vi "XLP80_Action_UpdateWriteB_newState.vi"(8 "err in":errorcluster, 10 "Function":string) -> (0 "err out":errorcluster)   [LabVIEW 2021]
uses:
  XLP80_FGlob/1886_FGlob_TDefs_Enum_FGlobItems.ctl
  XLP80_Globals/Globals_Settings_XLP80.vi
  XLP80_Globals/XLP80_Globals_Referenzen.vi
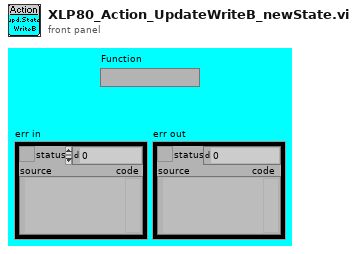
[diagram p1: front panel]
types:
  T1 = cluster{"Signal Name":string[], "Description":string[], "Unit":string[], "Default":dbl[], "Min":dbl[], "Max":dbl[], "Preconditions":bool[], "HV & Software":bool[], "Basis Funktion":bool[], "Power Management":bool[], "OperationMode":bool[], "Shutdown":bool[], "Alarm":bool[], "LogEnable":bool[]}
  T2 = typedef "1886_FGlob_TDefs_Enum_FGlobItems.ctl" = enum16{"Put one", "Put all", "Recall one", "Recall all"}
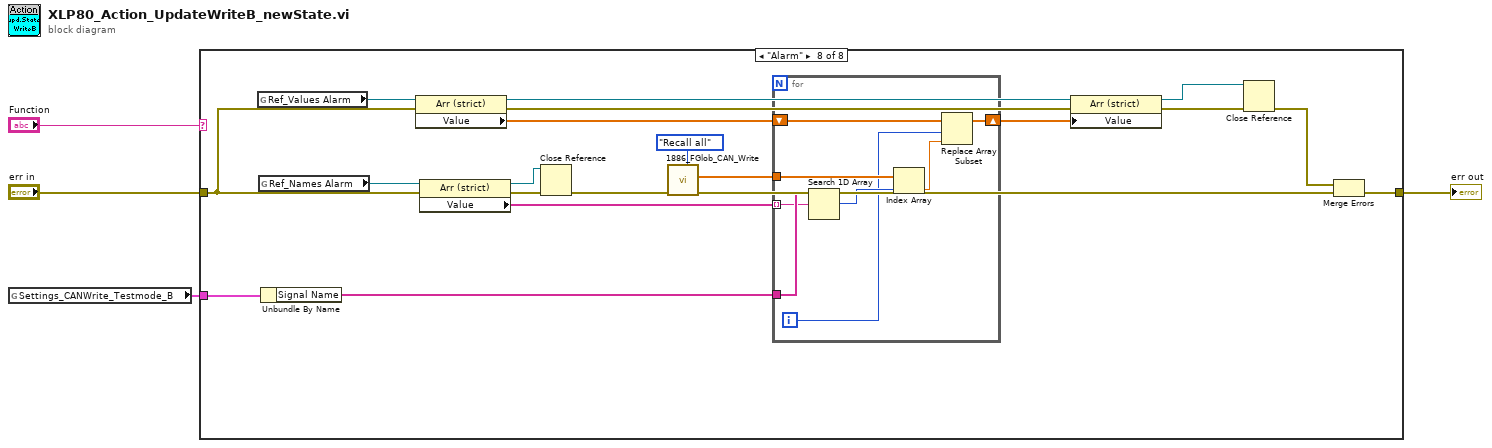
[diagram p0: block diagram]
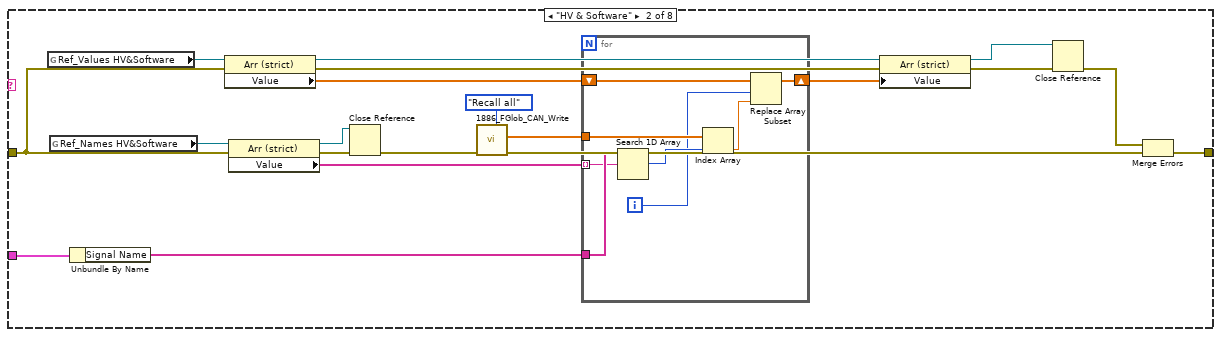
[diagram p3: hidden frame]
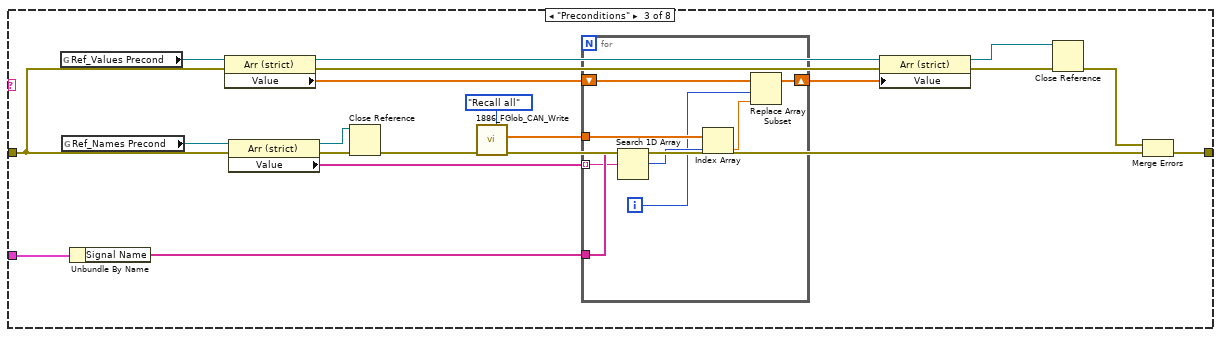
[diagram p4: hidden frame]
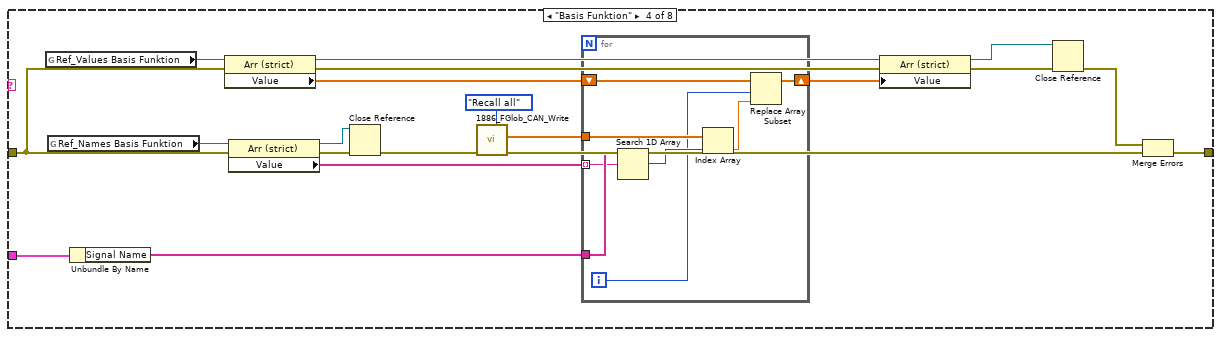
[diagram p5: hidden frame]
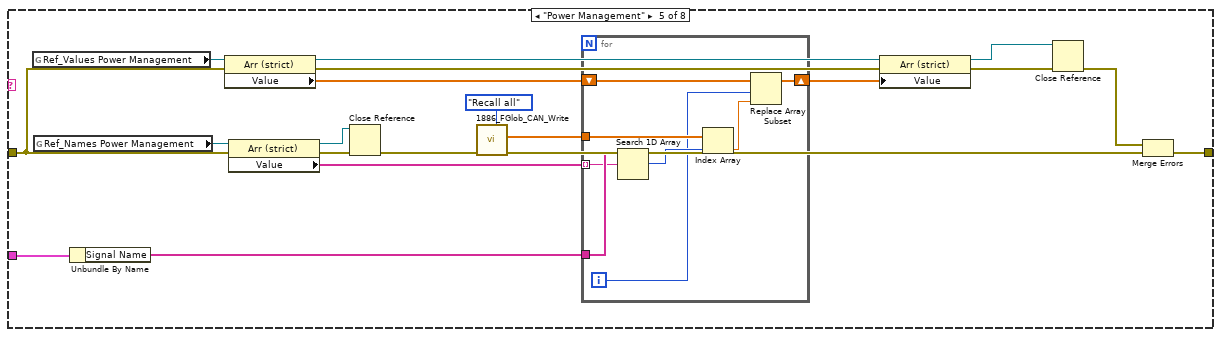
[diagram p6: hidden frame]
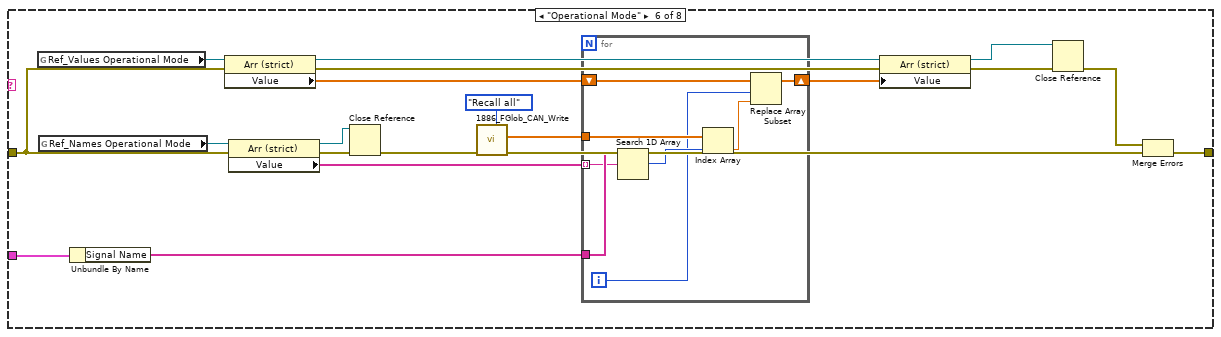
[diagram p7: hidden frame]
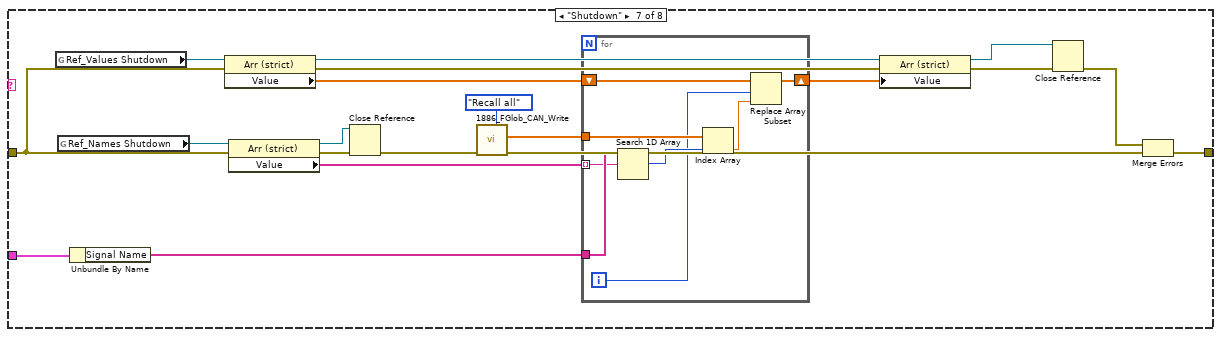
[diagram p8: hidden frame]
diagram:
  n1 = global read "Globals_Settings_XLP80.vi" "Settings_CANWrite_Testmode_B"() -> (w4:T1)
  n2 = case shown="\"Alarm\"" "Function" {
    tunnel: w4 -> [_ w19 w47 w75 w103 w131 w159 w187]
    tunnel: "err in" -> [w5 w18 w46 w74 w102 w130 w158 w186]
    tunnel: [w5 w21 w49 w77 w105 w133 w161 w189] -> w2
    frame Default {
    }
    frame "HV & Software" {
      n3 = global read "XLP80_Globals_Referenzen.vi" "Ref_Values HV&Software"() -> (w22:refnum<vi>)
      n4 = global read "XLP80_Globals_Referenzen.vi" "Ref_Names HV&Software"() -> (w23:refnum<vi>)
      n5 = Unbundle By Name(w19) -> ("Signal Name"=w15:string[])
      n6 = property class="Arr (strict)"(reference=w22, error in=w18) -> (reference out=w10:refnum<vi>, error out=w9:errorcluster, "Value"=w17:dbl[])
      n7 = property class="Arr (strict)"(reference=w23, error in=w18) -> (reference out=w24:refnum<vi>, error out=w25:errorcluster, "Value"=w16:string[])
      n8 = Close Reference(reference=w24, error in (no error)=w25) -> (error out=w14:errorcluster)
      n9 = call "1886_FGlob_CAN_Write.vi"("Function (Recall One)"=1886_FGlob_TDefs_Enum_FGlobItems."Recall all", "err in"=w14) -> ("err out"=w11:errorcluster, "AO Values OUT"=w12:dbl[])  [unwired: 7 in, 1 out]
      n10 = for {
        shift-right: [w26] -> w8
        shift-left: w17 -> [w31]
        tunnel: w16 -> [w32] mode=indexing
        tunnel: w15 -> [w33]
        tunnel: w12 -> [w30]
        i -> [w28]
        n11 = Search 1D Array(1D array=w33, element=w32) -> (index of element=w29:i32)  [unwired: 1 in]
        n12 = Index Array(array=w30, index=w29) -> (element=w27:dbl)
        n13 = Replace Array Subset(array=w31, new element=w27, index=w28) -> (w26:dbl[])
      }
      n14 = property class="Arr (strict)"(reference=w10, error in=w9, "Value"=w8) -> (reference out=w7:refnum<vi>, error out=w6:errorcluster)
      n15 = Close Reference(reference=w7, error in (no error)=w6) -> (error out=w20:errorcluster)
      n16 = Merge Errors(w20, w11) -> (w21:errorcluster)
    }
    frame "Preconditions" {
      n17 = global read "XLP80_Globals_Referenzen.vi" "Ref_Values Precond"() -> (w50:refnum<vi>)
      n18 = global read "XLP80_Globals_Referenzen.vi" "Ref_Names Precond"() -> (w51:refnum<vi>)
      n19 = Unbundle By Name(w47) -> ("Signal Name"=w43:string[])
      n20 = property class="Arr (strict)"(reference=w50, error in=w46) -> (reference out=w38:refnum<vi>, error out=w37:errorcluster, "Value"=w45:dbl[])
      n21 = property class="Arr (strict)"(reference=w51, error in=w46) -> (reference out=w52:refnum<vi>, error out=w53:errorcluster, "Value"=w44:string[])
      n22 = Close Reference(reference=w52, error in (no error)=w53) -> (error out=w42:errorcluster)
      n23 = call "1886_FGlob_CAN_Write.vi"("Function (Recall One)"=1886_FGlob_TDefs_Enum_FGlobItems."Recall all", "err in"=w42) -> ("err out"=w39:errorcluster, "AO Values OUT"=w40:dbl[])  [unwired: 7 in, 1 out]
      n24 = for {
        shift-right: [w54] -> w36
        shift-left: w45 -> [w59]
        tunnel: w44 -> [w60] mode=indexing
        tunnel: w43 -> [w61]
        tunnel: w40 -> [w58]
        i -> [w56]
        n25 = Search 1D Array(1D array=w61, element=w60) -> (index of element=w57:i32)  [unwired: 1 in]
        n26 = Index Array(array=w58, index=w57) -> (element=w55:dbl)
        n27 = Replace Array Subset(array=w59, new element=w55, index=w56) -> (w54:dbl[])
      }
      n28 = property class="Arr (strict)"(reference=w38, error in=w37, "Value"=w36) -> (reference out=w35:refnum<vi>, error out=w34:errorcluster)
      n29 = Close Reference(reference=w35, error in (no error)=w34) -> (error out=w48:errorcluster)
      n30 = Merge Errors(w48, w39) -> (w49:errorcluster)
    }
    frame "Basis Funktion" {
      n31 = global read "XLP80_Globals_Referenzen.vi" "Ref_Values Basis Funktion"() -> (w78:refnum<vi>)
      n32 = global read "XLP80_Globals_Referenzen.vi" "Ref_Names Basis Funktion"() -> (w79:refnum<vi>)
      n33 = Unbundle By Name(w75) -> ("Signal Name"=w71:string[])
      n34 = property class="Arr (strict)"(reference=w78, error in=w74) -> (reference out=w66:refnum<vi>, error out=w65:errorcluster, "Value"=w73:dbl[])
      n35 = property class="Arr (strict)"(reference=w79, error in=w74) -> (reference out=w80:refnum<vi>, error out=w81:errorcluster, "Value"=w72:string[])
      n36 = Close Reference(reference=w80, error in (no error)=w81) -> (error out=w70:errorcluster)
      n37 = call "1886_FGlob_CAN_Write.vi"("Function (Recall One)"=1886_FGlob_TDefs_Enum_FGlobItems."Recall all", "err in"=w70) -> ("err out"=w67:errorcluster, "AO Values OUT"=w68:dbl[])  [unwired: 7 in, 1 out]
      n38 = for {
        shift-right: [w82] -> w64
        shift-left: w73 -> [w87]
        tunnel: w72 -> [w88] mode=indexing
        tunnel: w71 -> [w89]
        tunnel: w68 -> [w86]
        i -> [w84]
        n39 = Search 1D Array(1D array=w89, element=w88) -> (index of element=w85:i32)  [unwired: 1 in]
        n40 = Index Array(array=w86, index=w85) -> (element=w83:dbl)
        n41 = Replace Array Subset(array=w87, new element=w83, index=w84) -> (w82:dbl[])
      }
      n42 = property class="Arr (strict)"(reference=w66, error in=w65, "Value"=w64) -> (reference out=w63:refnum<vi>, error out=w62:errorcluster)
      n43 = Close Reference(reference=w63, error in (no error)=w62) -> (error out=w76:errorcluster)
      n44 = Merge Errors(w76, w67) -> (w77:errorcluster)
    }
    frame "Power Management" {
      n45 = global read "XLP80_Globals_Referenzen.vi" "Ref_Values Power Management"() -> (w106:refnum<vi>)
      n46 = global read "XLP80_Globals_Referenzen.vi" "Ref_Names Power Management"() -> (w107:refnum<vi>)
      n47 = Unbundle By Name(w103) -> ("Signal Name"=w99:string[])
      n48 = property class="Arr (strict)"(reference=w106, error in=w102) -> (reference out=w94:refnum<vi>, error out=w93:errorcluster, "Value"=w101:dbl[])
      n49 = property class="Arr (strict)"(reference=w107, error in=w102) -> (reference out=w108:refnum<vi>, error out=w109:errorcluster, "Value"=w100:string[])
      n50 = Close Reference(reference=w108, error in (no error)=w109) -> (error out=w98:errorcluster)
      n51 = call "1886_FGlob_CAN_Write.vi"("Function (Recall One)"=1886_FGlob_TDefs_Enum_FGlobItems."Recall all", "err in"=w98) -> ("err out"=w95:errorcluster, "AO Values OUT"=w96:dbl[])  [unwired: 7 in, 1 out]
      n52 = for {
        shift-right: [w110] -> w92
        shift-left: w101 -> [w115]
        tunnel: w100 -> [w116] mode=indexing
        tunnel: w99 -> [w117]
        tunnel: w96 -> [w114]
        i -> [w112]
        n53 = Search 1D Array(1D array=w117, element=w116) -> (index of element=w113:i32)  [unwired: 1 in]
        n54 = Index Array(array=w114, index=w113) -> (element=w111:dbl)
        n55 = Replace Array Subset(array=w115, new element=w111, index=w112) -> (w110:dbl[])
      }
      n56 = property class="Arr (strict)"(reference=w94, error in=w93, "Value"=w92) -> (reference out=w91:refnum<vi>, error out=w90:errorcluster)
      n57 = Close Reference(reference=w91, error in (no error)=w90) -> (error out=w104:errorcluster)
      n58 = Merge Errors(w104, w95) -> (w105:errorcluster)
    }
    frame "Operational Mode" {
      n59 = global read "XLP80_Globals_Referenzen.vi" "Ref_Values Operational Mode"() -> (w134:refnum<vi>)
      n60 = global read "XLP80_Globals_Referenzen.vi" "Ref_Names Operational Mode"() -> (w135:refnum<vi>)
      n61 = Unbundle By Name(w131) -> ("Signal Name"=w127:string[])
      n62 = property class="Arr (strict)"(reference=w134, error in=w130) -> (reference out=w122:refnum<vi>, error out=w121:errorcluster, "Value"=w129:dbl[])
      n63 = property class="Arr (strict)"(reference=w135, error in=w130) -> (reference out=w136:refnum<vi>, error out=w137:errorcluster, "Value"=w128:string[])
      n64 = Close Reference(reference=w136, error in (no error)=w137) -> (error out=w126:errorcluster)
      n65 = call "1886_FGlob_CAN_Write.vi"("Function (Recall One)"=1886_FGlob_TDefs_Enum_FGlobItems."Recall all", "err in"=w126) -> ("err out"=w123:errorcluster, "AO Values OUT"=w124:dbl[])  [unwired: 7 in, 1 out]
      n66 = for {
        shift-right: [w138] -> w120
        shift-left: w129 -> [w143]
        tunnel: w128 -> [w144] mode=indexing
        tunnel: w127 -> [w145]
        tunnel: w124 -> [w142]
        i -> [w140]
        n67 = Search 1D Array(1D array=w145, element=w144) -> (index of element=w141:i32)  [unwired: 1 in]
        n68 = Index Array(array=w142, index=w141) -> (element=w139:dbl)
        n69 = Replace Array Subset(array=w143, new element=w139, index=w140) -> (w138:dbl[])
      }
      n70 = property class="Arr (strict)"(reference=w122, error in=w121, "Value"=w120) -> (reference out=w119:refnum<vi>, error out=w118:errorcluster)
      n71 = Close Reference(reference=w119, error in (no error)=w118) -> (error out=w132:errorcluster)
      n72 = Merge Errors(w132, w123) -> (w133:errorcluster)
    }
    frame "Shutdown" {
      n73 = global read "XLP80_Globals_Referenzen.vi" "Ref_Values Shutdown"() -> (w162:refnum<vi>)
      n74 = global read "XLP80_Globals_Referenzen.vi" "Ref_Names Shutdown"() -> (w163:refnum<vi>)
      n75 = Unbundle By Name(w159) -> ("Signal Name"=w155:string[])
      n76 = property class="Arr (strict)"(reference=w162, error in=w158) -> (reference out=w150:refnum<vi>, error out=w149:errorcluster, "Value"=w157:dbl[])
      n77 = property class="Arr (strict)"(reference=w163, error in=w158) -> (reference out=w164:refnum<vi>, error out=w165:errorcluster, "Value"=w156:string[])
      n78 = Close Reference(reference=w164, error in (no error)=w165) -> (error out=w154:errorcluster)
      n79 = call "1886_FGlob_CAN_Write.vi"("Function (Recall One)"=1886_FGlob_TDefs_Enum_FGlobItems."Recall all", "err in"=w154) -> ("err out"=w151:errorcluster, "AO Values OUT"=w152:dbl[])  [unwired: 7 in, 1 out]
      n80 = for {
        shift-right: [w166] -> w148
        shift-left: w157 -> [w171]
        tunnel: w156 -> [w172] mode=indexing
        tunnel: w155 -> [w173]
        tunnel: w152 -> [w170]
        i -> [w168]
        n81 = Search 1D Array(1D array=w173, element=w172) -> (index of element=w169:i32)  [unwired: 1 in]
        n82 = Index Array(array=w170, index=w169) -> (element=w167:dbl)
        n83 = Replace Array Subset(array=w171, new element=w167, index=w168) -> (w166:dbl[])
      }
      n84 = property class="Arr (strict)"(reference=w150, error in=w149, "Value"=w148) -> (reference out=w147:refnum<vi>, error out=w146:errorcluster)
      n85 = Close Reference(reference=w147, error in (no error)=w146) -> (error out=w160:errorcluster)
      n86 = Merge Errors(w160, w151) -> (w161:errorcluster)
    }
    frame "Alarm" {
      n87 = global read "XLP80_Globals_Referenzen.vi" "Ref_Values Alarm"() -> (w190:refnum<vi>)
      n88 = global read "XLP80_Globals_Referenzen.vi" "Ref_Names Alarm"() -> (w191:refnum<vi>)
      n89 = Unbundle By Name(w187) -> ("Signal Name"=w183:string[])
      n90 = property class="Arr (strict)"(reference=w190, error in=w186) -> (reference out=w178:refnum<vi>, error out=w177:errorcluster, "Value"=w185:dbl[])
      n91 = property class="Arr (strict)"(reference=w191, error in=w186) -> (reference out=w192:refnum<vi>, error out=w193:errorcluster, "Value"=w184:string[])
      n92 = Close Reference(reference=w192, error in (no error)=w193) -> (error out=w182:errorcluster)
      n93 = call "1886_FGlob_CAN_Write.vi"("Function (Recall One)"=1886_FGlob_TDefs_Enum_FGlobItems."Recall all", "err in"=w182) -> ("err out"=w179:errorcluster, "AO Values OUT"=w180:dbl[])  [unwired: 7 in, 1 out]
      n94 = for {
        shift-right: [w194] -> w176
        shift-left: w185 -> [w199]
        tunnel: w184 -> [w200] mode=indexing
        tunnel: w183 -> [w201]
        tunnel: w180 -> [w198]
        i -> [w196]
        n95 = Search 1D Array(1D array=w201, element=w200) -> (index of element=w197:i32)  [unwired: 1 in]
        n96 = Index Array(array=w198, index=w197) -> (element=w195:dbl)
        n97 = Replace Array Subset(array=w199, new element=w195, index=w196) -> (w194:dbl[])
      }
      n98 = property class="Arr (strict)"(reference=w178, error in=w177, "Value"=w176) -> (reference out=w175:refnum<vi>, error out=w174:errorcluster)
      n99 = Close Reference(reference=w175, error in (no error)=w174) -> (error out=w188:errorcluster)
      n100 = Merge Errors(w188, w179) -> (w189:errorcluster)
    }
  }
  "err out" <- w2
